vi "电流采样测试与校准.vi"() -> ()   [LabVIEW 2020]
uses:
  <vilib>/Utility/file.llb/Write Delimited Spreadsheet (string).vi
panel:
  in  "分流器条码":string
  in  "end":dbl=-400.0 caption="末端"
  in  "2700":refnum<visa-resource-name>="GPIB0::16::INSTR"
  in  "产品条码":string
  in  "产品型号":string="F020"
  out "表格控件":string[][](table) caption="测试结果"
  in  "start":dbl=400.0 caption="首端"
  in  "delta":dbl=-100.0
  in  "IT6512C":refnum<visa-resource-name>="GPIB0::16::INSTR"
  # "F020 分流器标定测试系统"
  # "仪器地址设置"
  # "产品信息"
  # "电流条件"
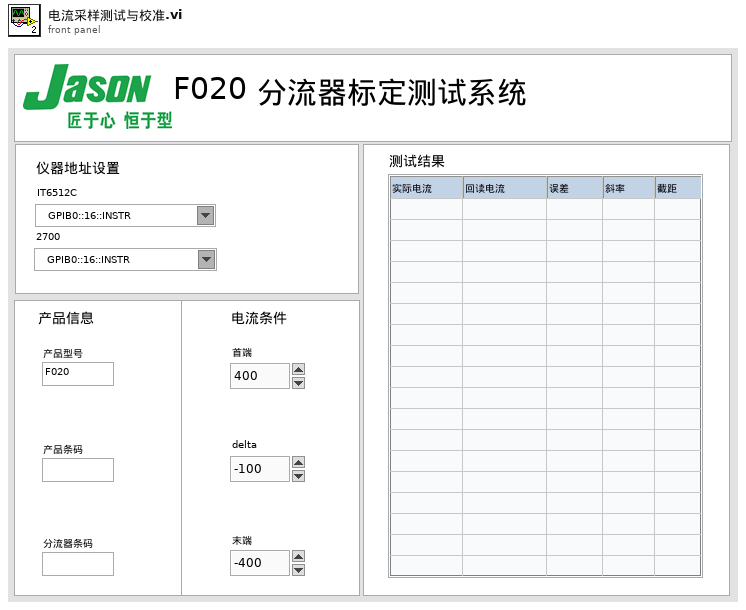
[diagram p1: front panel]
types:
  T1 = enum16{"open", "replace", "create", "open or create", "replace or create", "replace or create with confirmation"}
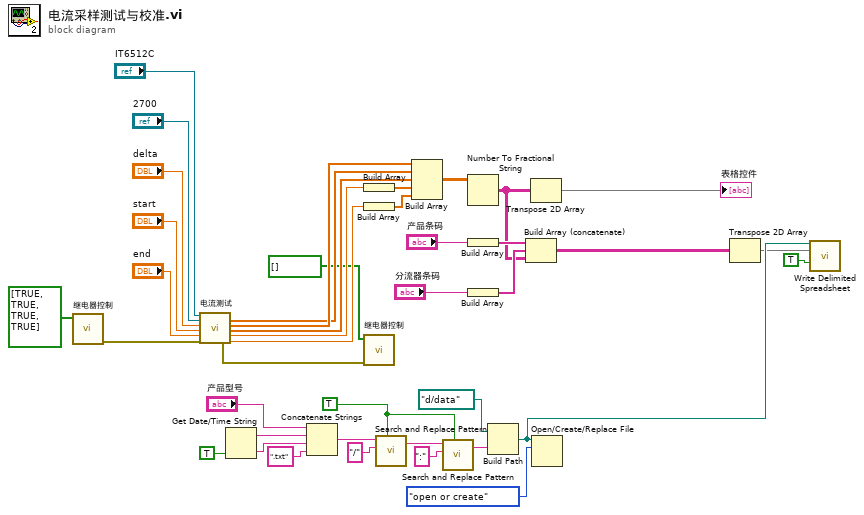
[diagram p0: block diagram]
diagram:
  w1 = TRUE ("replace all? (F)")
  n1 = call "继电器控制.vi"("继电器控制"=bool[] [TRUE, TRUE, TRUE, TRUE]) -> ("error out"=w4:errorcluster)  [unwired: 10 in]
  n2 = call "电流测试.vi"("IT6512C"="IT6512C", "2700"="2700", "delta"="delta", "start"="start", "end"="end", "error in (no error)"=w4) -> ("error out"=w2:errorcluster, "回读电流"=w36:dbl[], "输入电流"=w37:dbl[], "误差"=w35:dbl[], "斜率"=w23:dbl, "截距"=w22:dbl)  [unwired: 8 in]
  n3 = Get Date/Time String(want seconds? (F)=TRUE ("需要秒？(F)")) -> (date string=w32:string, time string=w31:string)  [unwired: 2 in]
  n4 = Concatenate Strings("产品型号", w32, w31, ".txt" ("字符串")) -> (w11:string)
  n5 = Build Array(w23) -> (w21:dbl[])
  n6 = Build Array(w22) -> (w20:dbl[])
  n7 = call "继电器控制.vi"("error in"=w2, "继电器控制"=bool[] []) -> ()  [unwired: 9 in, 1 out]
  n8 = call <vilib>:"Search and Replace Pattern.vi"("string"=w11, "regular expression (\"\")"="/" ("regular expression (\"\")"), "replace all? (F)"=w1) -> ("result string"=w9:string)  [unwired: 2 in, 1 out]
  n9 = Build Array(w37, w36, w35, w21, w20) -> (w26:dbl[][])
  n10 = call <vilib>:"Search and Replace Pattern.vi"("string"=w9, "regular expression (\"\")"=":" ("regular expression (\"\")"), "replace all? (F)"=w1) -> ("result string"=w6:string)  [unwired: 2 in, 1 out]
  n11 = Number To Fractional String(number=w26) -> (F-format string=w13:string[][])  [unwired: 3 in]
  n12 = Build Array("产品条码") -> (w17:string[])
  n13 = Build Array("分流器条码") -> (w15:string[])
  n14 = Build Path(base path=path "d:/data" ("基路径"), name or relative path=w6) -> (appended path=w28:path)
  n15 = Build Array (concatenate)(w17, w15, w13) -> (w14:string[][])
  n16 = Transpose 2D Array(2D array=w13) -> (transposed array=→"表格控件":string[][])
  n17 = Open/Create/Replace File(file path (use dialog)=w28, operation (0:open)=T1."open or create" ("操作(0:open)")) -> ()  [unwired: 4 in, 3 out]
  n18 = Transpose 2D Array(2D array=w14) -> (transposed array=w24:string[][])
  n19 = call-poly <vilib>:"Write Delimited Spreadsheet.vi"("file path (dialog if empty)"=w28, "2D data"=w24, "append to file? (new file:F)"=TRUE) -> ()  [unwired: 11 in, 2 out]
